vi "Exit.vi"   [LabVIEW 2015]
uses:
  lv64_eventdriven/board.vis/ESLSCDLL.dll
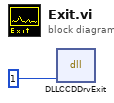
[diagram p0: block diagram]
diagram:
  n1 = dll-call lib="C:/ENTW/PCIE/64bit/lv64/lv64_eventdriven/board.vis/ESLSCDLL.dll" fn="DLLCCDDrvExit"("drv"=u32 1) -> ()  [unwired: 5 in, 2 out]
